vi "Default Scatter Property.vi"(11 "Plot ID":i32) -> (3 "Default Property":T1={"General Property"={"Plot Name"="", "Coordinate System"=enum."Cartesian", "Opacity"=0.0}, "Projection Property"={"Draw XY"=FALSE, "Draw YZ"=FALSE, "Draw XZ"=FALSE}, "Plot Property"={"Sprite Type"=enum."Empty Square", "Point Size"=0.0, "Color Ramp Cluster"={"Color Ramp Style"=enum."None", "Color Ramp Array"=[16711934, 393471, 57855, 4390754, 16449346, 16744722, 16711680], "Color Ramp Index"=[45, 91, 133, 175, 219, 255], "Interpolate?"=FALSE, "Logarithm?"=FALSE}}})   [LabVIEW 2017, in "3D Scatter.lvclass"]
uses:
  <vilib>/Math Plots/3D Math Plots/3D Scatter/3D Scatter/3D Scatter.lvclass
  <vilib>/Math Plots/3D Math Plots/3D Scatter/3D Scatter/Typedef/3D Scatter Property.ctl
  <vilib>/Math Plots/3D Math Plots/3D Plot/3D Plot/Typedef/Sprite Type.ctl
  <vilib>/Math Plots/3D Math Plots/3D Plot/3D Plot/Typedef/Color Ramp Cluster.ctl
  <vilib>/Math Plots/3D Math Plots/3D Plot/3D Plot/3D Plot.lvclass
panel:
  in  "Name Prefix":string="Plot "
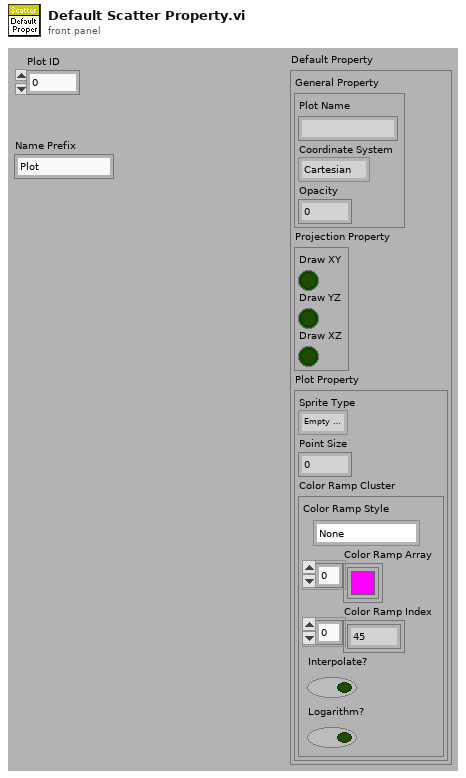
[diagram p1: front panel]
types:
  T1 = typedef "3D Scatter.lvclass/3D Scatter Property.ctl" = cluster{"General Property":cluster{"Plot Name":string, "Coordinate System":enum16{"Cartesian", "Cylindrical", "Spherical"}, "Opacity":sgl}, "Projection Property":cluster{"Draw XY":bool, "Draw YZ":bool, "Draw XZ":bool}, "Plot Property":cluster{"Sprite Type":T2, "Point Size":sgl, "Color Ramp Cluster":T3}}
  T2 = typedef "3D Plot.lvclass/Sprite Type.ctl" = enum16{"None", "Empty Square", "Solid Square", "Empty Diamond", "Solid Diamond", "Empty Circle", "Solid Circle", "Asterisk", "Bold X", "Wireframe Sphere", "Solid Sphere", "Wireframe Cube", "Solid Cube"}
  T3 = typedef "3D Plot.lvclass/Color Ramp Cluster.ctl" = cluster{"Color Ramp Style":enum16{"None", "Shaded", "Color spectrum", "Grey scale", "Custom"}, "Color Ramp Array":u32[], "Color Ramp Index":i32[], "Interpolate?":bool, "Logarithm?":bool}
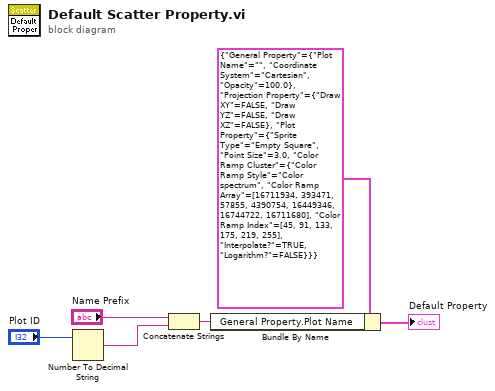
[diagram p0: block diagram]
diagram:
  n1 = Number To Decimal String(number="Plot ID") -> (decimal integer string=w6:string)  [unwired: 1 out]
  n2 = Concatenate Strings("Name Prefix", w6) -> (w3:string)
  n3 = Bundle By Name(cluster=T1 {"General Property"={"Plot Name"="", "Coordinate System"=enum."Cartesian", "Opacity"=100.0}, "Projection Property"={"Draw XY"=FALSE, "Draw YZ"=FALSE, "Draw XZ"=FALSE}, "Plot Property"={"Sprite Type"=enum."Empty Square", "Point Size"=3.0, "Color Ramp Cluster"={"Color Ramp Style"=enum."Color spectrum", "Color Ramp Array"=[16711934, 393471, 57855, 4390754, 16449346, 16744722, 16711680], "Color Ramp Index"=[45, 91, 133, 175, 219, 255], "Interpolate?"=TRUE, "Logarithm?"=FALSE}}} ("new element/subarray"), "General Property.Plot Name"=w3) -> (→"Default Property":T1)
